vi "Open.vi"(7 "Config data in":variant, 8 "error in (no error)":errorcluster, 9 "Timeout (ms)":u32=3000, 10 "VISA session":refnum<visa-resource-name>="TCPIP::146.201.232.88::7180::SOCKET", 11 "PS Driver AMI4xx.lvlib:PS Driver AMI4xx.lvclass in":refnum<class "PS Driver AMI4xx.lvclass">) -> (0 "error out":errorcluster, 1 "Config data out":variant, 2 "dup VISA Session":refnum<visa-resource-name>, 3 "PS Driver AMI4xx.lvlib:PS Driver AMI4xx.lvclass out":refnum<class "PS Driver AMI4xx.lvclass">)   [LabVIEW 2019, in "PS Driver.lvlib" / "PS Driver AMI4xx.lvclass"]
uses:
  PS Driver AMI4xx.lvclass
  PS Driver.lvclass
  PS Driver with Persistence.lvclass
  C:/Users/coniglio/Documents/SCM_PS_AF/PS Driver/PS Driver with Persistence.lvclass
  C:/Users/coniglio/Documents/SCM_PS_AF/PS Driver/PS Driver.lvclass
panel:
  out "IDN string":string
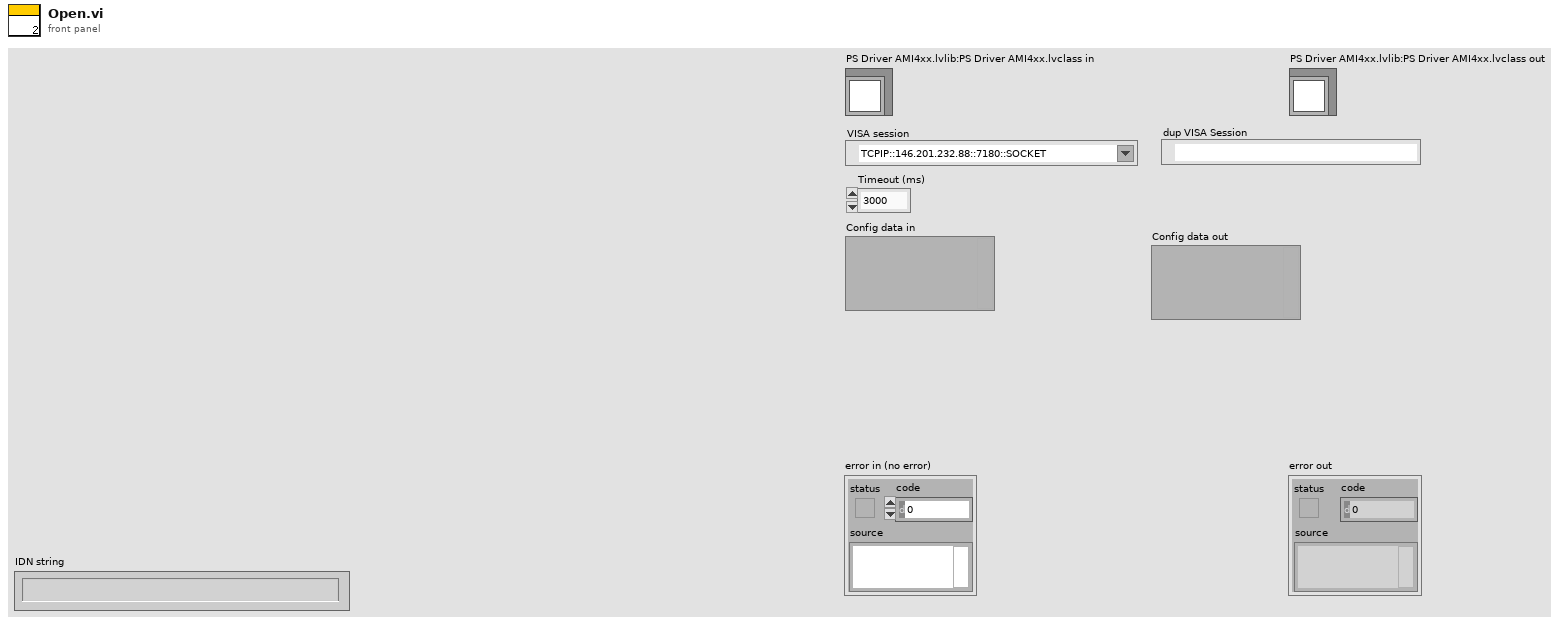
[diagram p1: front panel]
types:
  T1 = cluster{"INI key name":string, "Configuration command":string}[]
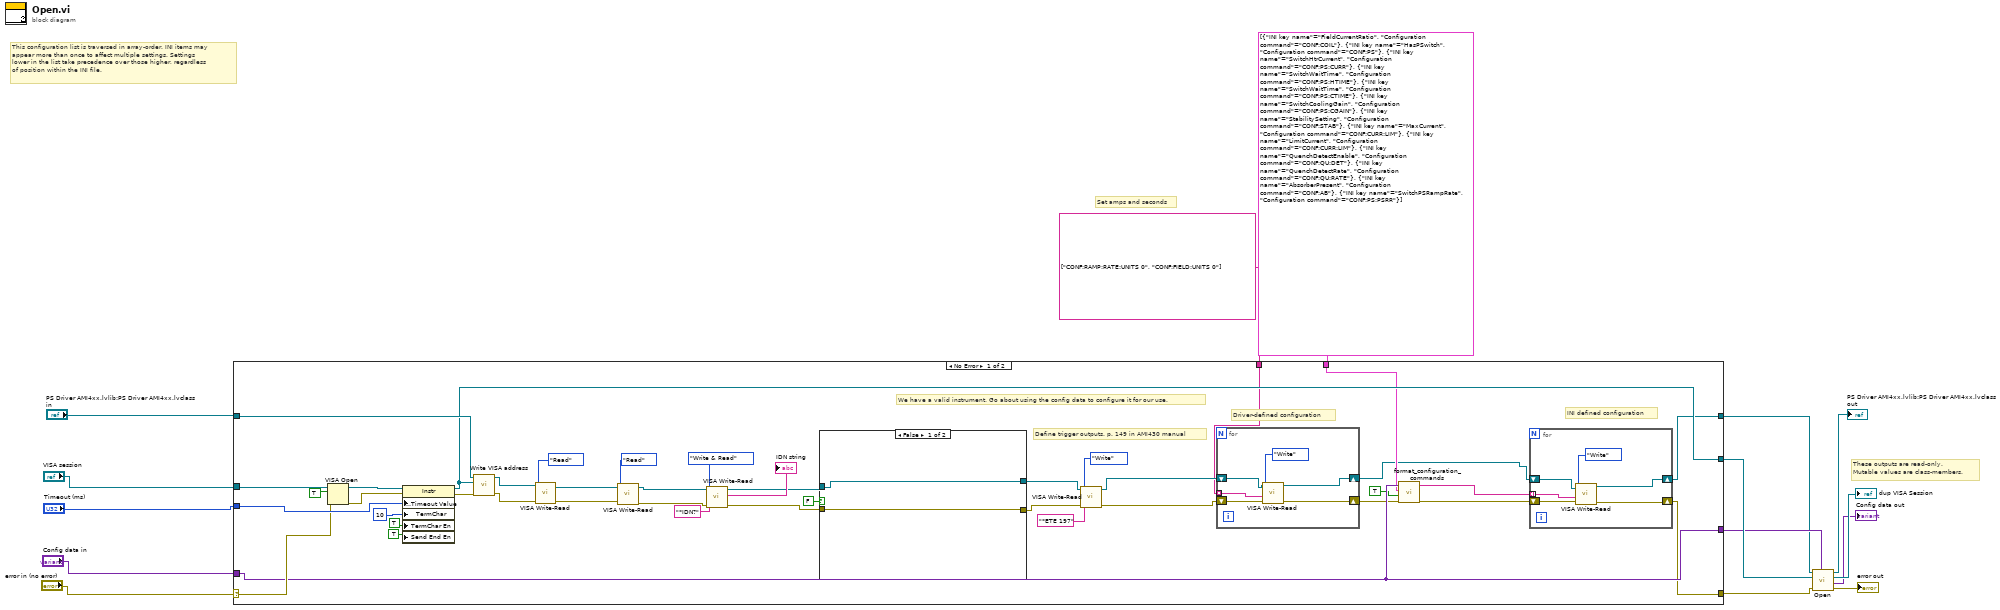
[diagram p0: block diagram]
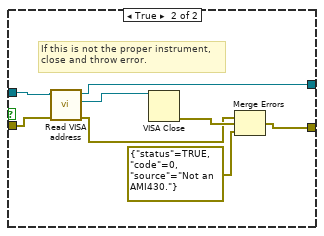
[diagram p2: hidden frame]
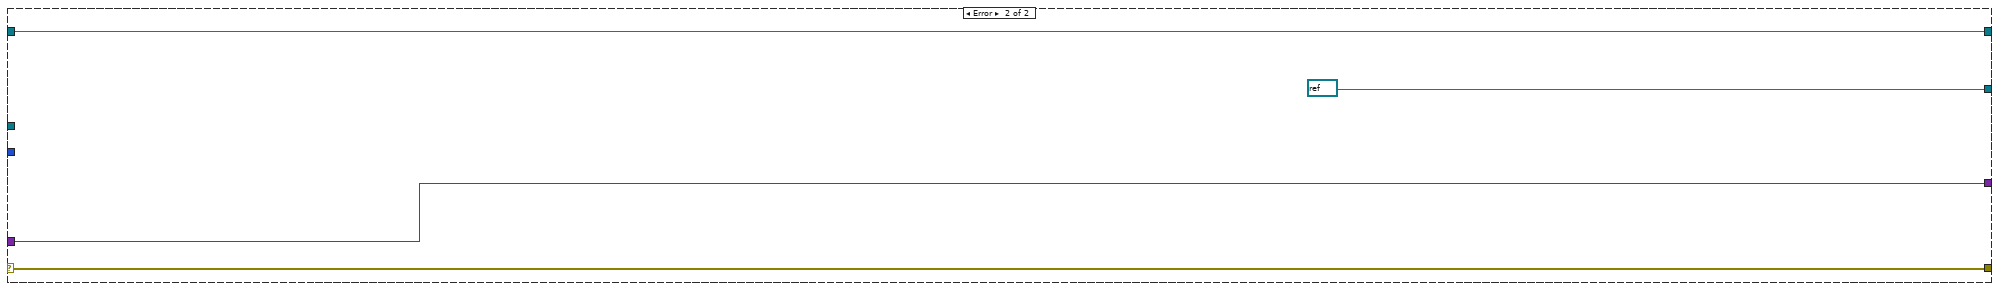
[diagram p3: hidden frame]
diagram:
  # "Set amps and seconds"
  # "These outputs are read-only.\nMutable values are class-members."
  # "This configuration list is traversed in array-order. INI items may\nappear more than once to affect multiple settings. Settings\nlower in the list take precedence over those higher, regardless\nof position within the INI file."
  n1 = case shown="No Error" "error in (no error)" {
    selector: "error in (no error)" -> [w49 w83]
    tunnel: [w21 w83] -> w14
    tunnel: [w22 w82] -> w11
    tunnel: "PS Driver AMI4xx.lvlib:PS Driver AMI4xx.lvclass in" -> [w35 w82]
    tunnel: "VISA session" -> [w51 _]
    tunnel: "Timeout (ms)" -> [w50 _]
    tunnel: "Config data in" -> [w27 w80]
    tunnel: [w28 refnum<visa-resource-name> refnum ("dup VISA Session")] -> w15
    tunnel: [w27 w80] -> w12
    tunnel: T1 [{"INI key name"="FieldCurrentRatio", "Configuration command"="CONF:COIL"}, {"INI key name"="HasPSwitch", "Configuration command"="CONF:PS"}, {"INI key name"="SwitchHtrCurrent", "Configuration command"="CONF:PS:CURR"}, {"INI key name"="SwitchWaitTime", "Configuration command"="CONF:PS:HTIME"}, {"INI key name"="SwitchWaitTime", "Configuration command"="CONF:PS:CTIME"}, {"INI key name"="SwitchCoolingGain", "Configuration command"="CONF:PS:CGAIN"}, {"INI key name"="StabilitySetting", "Configuration command"="CONF:STAB"}, {"INI key name"="MaxCurrent", "Configuration command"="CONF:CURR:LIM"}, {"INI key name"="LimitCurrent", "Configuration command"="CONF:CURR:LIM"}, {"INI key name"="QuenchDetectEnable", "Configuration command"="CONF:QU:DET"}, {"INI key name"="QuenchDetectRate", "Configuration command"="CONF:QU:RATE"}, {"INI key name"="AbsorberPresent", "Configuration command"="CONF:AB"}, {"INI key name"="SwitchPSRampRate", "Configuration command"="CONF:PS:PSRR"}] -> [w26 _]
    tunnel: string[] ["CONF:RAMP:RATE:UNITS 0", "CONF:FIELD:UNITS 0"] -> [w16 _]
    frame No Error {
      # "Driver-defined configuration"
      # "INI defined configuration"
      # "Define trigger outputs. p. 149 in AMI430 manual"
      # "We have a valid instrument. Go about using the config data to configure it for our use."
      n2 = VISA Open(duplicate session (F)=TRUE, error in (no error)=w49, VISA resource name=w51) -> (VISA resource name=w57:refnum<visa-resource-name>, error out=w55:errorcluster)  [unwired: 2 in]
      n3 = property class="Instr"(reference=w57, error in=w55, "General Settings:Timeout Value"=w50, "TermChar"=u8 10 ("Message Based Settings:Termination Character"), "TermChar En"=TRUE ("Message Based Settings:Termination Character Enable"), "Send End En"=TRUE ("Message Based Settings:Send End Enable")) -> (reference out=w28:refnum<visa-resource-name>, error out=w36:errorcluster)
      n4 = call "Write VISA address.vi"("error in (no error)"=w36, "VISA address"=w28, "PS Driver in"=w35) -> ("error out"=w33:errorcluster, "PS Driver out"=w34:refnum<class "PS Driver AMI4xx.lvclass">)  [unwired: 7 in]
      n5 = call "VISA Write-Read.vi"("error in (no error)"=w33, "Action"=enum16{"Write", "Read", "Write & Read"}."Read", "PS Driver.lvlib:PS Driver AMI4xx.lvclass"=w34) -> ("error out"=w37:errorcluster, "PS Driver.lvlib:PS Driver AMI4xx.lvclass out"=w38:refnum<class "PS Driver AMI4xx.lvclass">)  [unwired: 5 in, 2 out]
      n6 = call "VISA Write-Read.vi"("error in (no error)"=w37, "Action"=enum16{"Write", "Read", "Write & Read"}."Read", "PS Driver.lvlib:PS Driver AMI4xx.lvclass"=w38) -> ("error out"=w39:errorcluster, "PS Driver.lvlib:PS Driver AMI4xx.lvclass out"=w40:refnum<class "PS Driver AMI4xx.lvclass">)  [unwired: 5 in, 2 out]
      n7 = call "VISA Write-Read.vi"("error in (no error)"=w39, "Command String"="*IDN?", "Action"=enum16{"Write", "Read", "Write & Read"}."Write & Read", "PS Driver.lvlib:PS Driver AMI4xx.lvclass"=w40) -> ("error out"=w43:errorcluster, "Response string"=→"IDN string":string, "PS Driver.lvlib:PS Driver AMI4xx.lvclass out"=w41:refnum<class "PS Driver AMI4xx.lvclass">)  [unwired: 4 in, 1 out]
      n8 = case shown="False" FALSE {
        tunnel: w43 -> [w71 w74]
        tunnel: [w71 w77] -> w30
        tunnel: [w70 w75] -> w29
        tunnel: w41 -> [w70 w72]
        frame False {
        }
        frame True {
          # "If this is not the proper instrument,\nclose and throw error."
          n9 = call "Read VISA address.vi"("error in (no error)"=w74, "PS Driver in"=w72) -> ("error out"=w73:errorcluster, "VISA address"=w76:refnum<visa-resource-name>, "PS Driver out"=w75:refnum<class "PS Driver AMI4xx.lvclass">)  [unwired: 7 in]
          n10 = VISA Close(VISA resource name=w76) -> (error out=w79:errorcluster)  [unwired: 1 in]
          n11 = Merge Errors(w73, w79, errorcluster {"status"=TRUE, "code"=0, "source"="Not an AMI430."} ("error IO")) -> (w77:errorcluster)
        }
      }
      n12 = call "VISA Write-Read.vi"("error in (no error)"=w30, "Command String"="*ETE 197", "Action"=enum16{"Write", "Read", "Write & Read"}."Write", "PS Driver.lvlib:PS Driver AMI4xx.lvclass"=w29) -> ("error out"=w19:errorcluster, "PS Driver.lvlib:PS Driver AMI4xx.lvclass out"=w20:refnum<class "PS Driver AMI4xx.lvclass">)  [unwired: 4 in, 2 out]
      n13 = for {
        shift-right: [w58] -> w18
        shift-left: w19 -> [w61]
        shift-right: [w59] -> w17
        shift-left: w20 -> [w62]
        tunnel: w16 -> [w60] mode=indexing
        n14 = call "VISA Write-Read.vi"("error in (no error)"=w61, "Command String"=w60, "Action"=enum16{"Write", "Read", "Write & Read"}."Write", "PS Driver.lvlib:PS Driver AMI4xx.lvclass"=w62) -> ("error out"=w58:errorcluster, "PS Driver.lvlib:PS Driver AMI4xx.lvclass out"=w59:refnum<class "PS Driver AMI4xx.lvclass">)  [unwired: 4 in, 2 out]
      }
      n15 = call "format_configuration_commands.vi"("error in (no error)"=w18, "True/false to 0/1?"=TRUE, "Configuration editables"=w26, "Config data in"=w27) -> ("error out"=w24:errorcluster, "Configuration commands"=w23:string[])  [unwired: 6 in]
      n16 = for {
        shift-right: [w64] -> w21
        shift-left: w24 -> [w67]
        shift-right: [w65] -> w22
        shift-left: w17 -> [w68]
        tunnel: w23 -> [w66] mode=indexing
        n17 = call "VISA Write-Read.vi"("error in (no error)"=w67, "Command String"=w66, "Action"=enum16{"Write", "Read", "Write & Read"}."Write", "PS Driver.lvlib:PS Driver AMI4xx.lvclass"=w68) -> ("error out"=w64:errorcluster, "PS Driver.lvlib:PS Driver AMI4xx.lvclass out"=w65:refnum<class "PS Driver AMI4xx.lvclass">)  [unwired: 4 in, 2 out]
      }
    }
    frame Error {
    }
  }
  n18 = call-parent "Open.vi"("Config data in"=w12, "error in (no error)"=w14, "VISA session"=w15, "PS Driver.lvlib:PS Driver.lvclass in"=w11) -> ("error out"=→"error out":errorcluster, "Config data out"=→"Config data out":variant, "dup VISA Session"=→"dup VISA Session":refnum<visa-resource-name>, "PS Driver.lvlib:PS Driver.lvclass out"=→"PS Driver AMI4xx.lvlib:PS Driver AMI4xx.lvclass out":refnum<class "PS Driver AMI4xx.lvclass">)  [unwired: 4 in]
